vi "GOOP_XControl_Item_Interface.vi"() -> (3 "InterfaceTable":T1)   [LabVIEW 2020]
uses:
  <resource>/Framework/Providers/API/Item_Interface.ctl
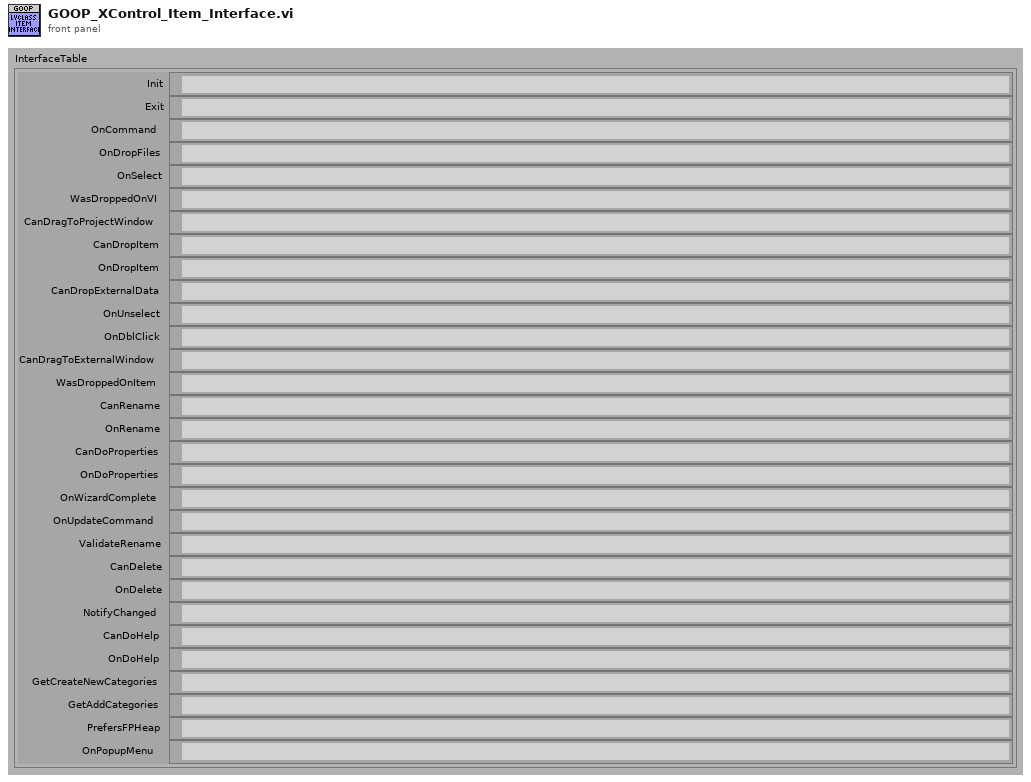
[diagram p1: front panel]
types:
  T1 = typedef "Item_Interface.ctl" = cluster{"Init":path, "Exit":path, "OnCommand":path, "OnDropFiles":path, "OnSelect":path, "WasDroppedOnVI":path, "CanDragToProjectWindow":path, "CanDropItem":path, "OnDropItem":path, "CanDropExternalData":path, "OnUnselect":path, "OnDblClick":path, "CanDragToExternalWindow":path, "WasDroppedOnItem":path, "CanRename":path, "OnRename":path, "CanDoProperties":path, "OnDoProperties":path, "OnWizardComplete":path, "OnUpdateCommand":path, "ValidateRename":path, "CanDelete":path, "OnDelete":path, "NotifyChanged":path, "CanDoHelp":path, "OnDoHelp":path, "GetCreateNewCategories":path, "GetAddCategories":path, "PrefersFPHeap":path, "OnPopupMenu":path}
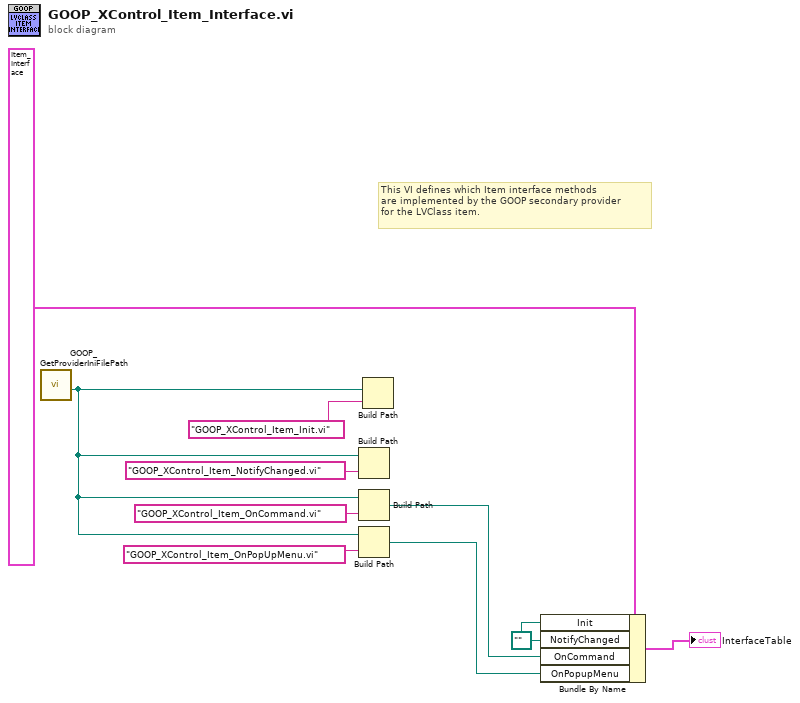
[diagram p0: block diagram]
diagram:
  w1 = path "" ("NotifyChanged")
  # "This VI defines which Item interface methods \nare implemented by the GOOP secondary provider \nfor the LVClass item."
  n1 = call "GOOP_GetProviderIniFilePath.vi"() -> ("ProviderMainFolder"=w5:path)  [unwired: 10 in, 1 out]
  n2 = Build Path(base path=w5, name or relative path="GOOP_XControl_Item_NotifyChanged.vi") -> ()  [unwired: 1 out]
  n3 = Build Path(base path=w5, name or relative path="GOOP_XControl_Item_OnCommand.vi") -> (appended path=w3:path)
  n4 = Build Path(base path=w5, name or relative path="GOOP_XControl_Item_OnPopUpMenu.vi") -> (appended path=w2:path)
  n5 = Build Path(base path=w5, name or relative path="GOOP_XControl_Item_Init.vi") -> ()  [unwired: 1 out]
  n6 = Bundle By Name(cluster=T1 {"Init"=path "", "Exit"=path "", "OnCommand"=path "", "OnDropFiles"=path "", "OnSelect"=path "", "WasDroppedOnVI"=path "", "CanDragToProjectWindow"=path "", "CanDropItem"=path "", "OnDropItem"=path "", "CanDropExternalData"=path "", "OnUnselect"=path "", "OnDblClick"=path "", "CanDragToExternalWindow"=path "", "WasDroppedOnItem"=path "", "CanRename"=path "", "OnRename"=path "", "CanDoProperties"=path "", "OnDoProperties"=path "", "OnWizardComplete"=path "", "OnUpdateCommand"=path "", "ValidateRename"=path "", "CanDelete"=path "", "OnDelete"=path "", "NotifyChanged"=path "", "CanDoHelp"=path "", "OnDoHelp"=path "", "GetCreateNewCategories"=path "", "GetAddCategories"=path "", "PrefersFPHeap"=path "", "OnPopupMenu"=path ""} ("InterfaceTable"), "Init"=w1, "NotifyChanged"=w1, "OnCommand"=w3, "OnPopupMenu"=w2) -> (→"InterfaceTable":T1)
